vi "Receive Data Packet.vi"(8 "error in":errorcluster, 10 "Timeout (60000ms)":i32=60000, 11 "connection ID":refnum<k5>) -> (0 "error out":errorcluster, 1 "Packet #":u8, 2 "TCP/IP Data":u8[](array[numeric]), 3 "connection ID out":refnum<k5>)   [LabVIEW 2014, in "hse-db.lvlib" / "MySQL (TCP).lvlib"]
uses:
  MySQL (TCP).lvlib
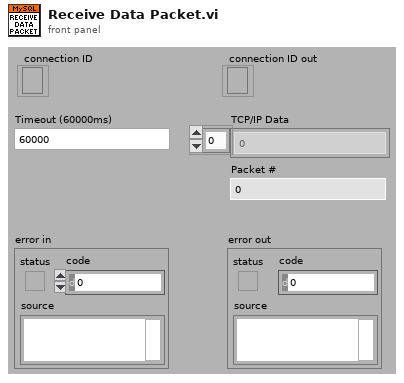
[diagram p1: front panel]
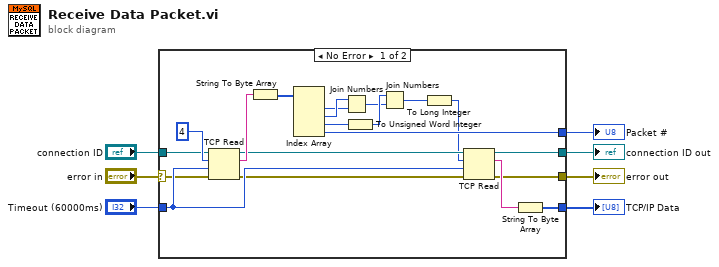
[diagram p0: block diagram]
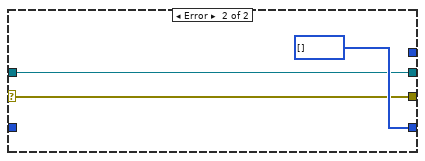
[diagram p2: hidden frame]
diagram:
  n1 = case shown="No Error" "error in" {
    selector: "error in" -> [w14 w28]
    tunnel: [w27 w29] -> w7
    tunnel: "Timeout (60000ms)" -> [w26 _]
    tunnel: "connection ID" -> [w16 w29]
    tunnel: [w12 w28] -> w4
    tunnel: [w13 u8[] [] ("unsigned byte array")] -> w3
    tunnel: [w10 _] -> w1
    frame No Error {
      n2 = TCP Read(connection ID=w16, bytes to read=4, error in (no error)=w14, 9:w26) -> (connection ID out=w11:refnum<k5>, data out=w19:string, error out=w18:errorcluster)  [unwired: 1 in]
      n3 = String To Byte Array(string=w19) -> (unsigned byte array=w20:u8[])
      n4 = Index Array(array=w20) -> (element #1=w21:u8, element #2=w22:u8, element #3=w25:u8, element #4=w10:u8)  [unwired: 4 in]
      n5 = Join Numbers(hi=w22, lo=w21) -> ((hi.lo)=w23:u16)
      n6 = To Unsigned Word Integer(number=w25) -> (unsigned 16bit integer=w24:u16)
      n7 = Join Numbers(hi=w24, lo=w23) -> ((hi.lo)=w9:u32)
      n8 = To Long Integer(number=w9) -> (32bit integer=w8:i32)
      n9 = TCP Read(connection ID=w11, bytes to read=w8, error in (no error)=w18, 9:w26) -> (connection ID out=w27:refnum<k5>, data out=w15:string, error out=w12:errorcluster)  [unwired: 1 in]
      n10 = String To Byte Array(string=w15) -> (unsigned byte array=w13:u8[])
    }
    frame Error {
    }
  }
  "connection ID out" <- w7
  "error out" <- w4
  "TCP/IP Data" <- w3
  "Packet #" <- w1
